vi "Actor Core.vi"(8 "error in":errorcluster, 11 "RecipeEditor in":refnum<class "RecipeEditor.lvclass">) -> (0 "error out":errorcluster, 3 "Actor out":refnum<class "Actor.lvclass">)   [LabVIEW 2024, in "RED Actor.lvlib" / "RecipeEditor.lvclass"]
doc: "(<B>Filename</B>: Actor Framework.lvlib:Actor.lvclass:Actor Core.vi)\n\nReceives messages to the actor, reacts to them, and initiates any error handling that may shut the actor down.\n\nDescendant classes may override this VI to append parallel tasks for the actor to complete while it handles messages. Overrides use the Call Parent Method node."
uses:
  RecipeEditor.lvclass
  C:/Program Files (x86)/National Instruments/LabVIEW 2024/vi.lib/ActorFramework/Actor/Actor.lvclass
  <vilib>/ActorFramework/Actor/Actor.lvclass
  Recipe.ctl
  Setting.ctl
  RedUiStatus.ctl
  RedFunc.ctl
  RecipeEditor.lvclass/RecipeEditor.ctl
  <vilib>/ActorFramework/Actor/Actor.lvclass/Actor.ctl
  <vilib>/ActorFramework/Message Enqueuer/Message Enqueuer.lvclass/Message Enqueuer.ctl
  <vilib>/ActorFramework/Message Enqueuer/Init from Existing Queue.vi
  <vilib>/ActorFramework/Message Enqueuer/Enqueue.vi
  <vilib>/ActorFramework/Stop Msg/Stop Msg.lvclass
  C:/Program Files (x86)/National Instruments/LabVIEW 2024/vi.lib/ActorFramework/Message/Message.lvclass
  Global Variables.vi
  <vilib>/ActorFramework/Message Priority Queue/Priority Enqueue.vi
  <vilib>/ActorFramework/Message Enqueuer/Message Enqueuer.lvclass
panel:
  in  "ExitEdit Button":bool
  out "UIStatus":T1
  in  "Setting Button":bool
  in  "Exit Button":bool
  in  "Save Button":bool
  in  "Upload Button":bool
  in  "Tab Control":enum32{"Recipe", "SystemSetting"}(tab)
  out "DriveWaveform":waveform(dbl)(graph)
  out "LoadWaveform":waveform(dbl)(graph)
  in  "RcpContent":T2={"LoadSide"={"LoadType"=enum."11kW Servo Motor", "LoadMode"=enum."Sin Wave", "LoadValue"=0.0, "PID"={"NP"=0.0, "NI"=0.0, "ND"=0.0, "NPS"="A", "NIS"="A", "NDS"="A"}, "SinWaveFormat"={"Crest"=0.0, "Trugh"=0.0, "Period"=0.0}}, "DriveSide"={"TestSpeed"=0.0, "SinWaveTorqueOutput"=FALSE, "SinWaveFormat"={"Crest"=0.0, "Trugh"=0.0, "Period"=0.0}}} {"DriveSide"."SinWaveFormat"."Period" min=0.0 max=99.0 format="%#.2f"; "DriveSide"."SinWaveFormat"."Trugh" min=0.0 max=99.0 step=1.0 format="%#.2f"; "DriveSide"."SinWaveFormat"."Crest" min=0.0 max=99.0 format="%#.2f"; "DriveSide"."TestSpeed" format="%#_2f"; "LoadSide"."SinWaveFormat"."Period" min=0.0 max=99.0 format="%#.2f"; "LoadSide"."SinWaveFormat"."Trugh" min=0.0 max=99.0 step=1.0 format="%#.2f"; "LoadSide"."SinWaveFormat"."Crest" min=0.0 max=99.0 format="%#.2f"; "LoadSide"."PID"."ND" min=0.0 max=99.0 format="%#.2f"; "LoadSide"."PID"."NI" min=0.0 max=99.0 step=1.0 format="%#.2f"; "LoadSide"."PID"."NP" min=0.0 max=99.0 format="%#.2f"; "LoadSide"."LoadValue" format="%#_2f"}
  in  "Search Button":bool
  in  "SearchingRcp":string
  in  "RecipeList":i32(listbox) caption="參數列表(*.rcp)"
  in  "RecipeFolder":path caption="參數資料夾路徑"
  in  "ButtonContainer":enum32{"Page 1", "Page 2"}(tab)
  in  "Add Button":bool
  in  "Remove Button":bool
  in  "Copy Button":bool
  in  "Modify Button":bool
  in  "TQCalib":bool
  in  "Setting":T3={"TorqueSensor"={"Interface"="", "Read Unit"=enum."Kg.cm", "Encoder"=0, "Torque Filter"=0, "Max Torque"=2.0, "Max Power"=50.0, "Max Speed"=50.0, "Scale Factor CW"=2.0, "Scale Factor CCW"=2.0, "Scale Factor Zero"=2.0}, "DC-1000"={"Interface"=enum."AD-1"}, "ServoMotor"={"Interface"=enum."AD-1"}} {"TorqueSensor"."Scale Factor Zero" format="%#.6f"; "TorqueSensor"."Scale Factor CCW" format="%#.6f"; "TorqueSensor"."Scale Factor CW" format="%#.6f"; "TorqueSensor"."Torque Filter" items=["OFF", "10Hz", "25Hz", "50Hz", "3Hz", "2Hz", "1Hz"]; "TorqueSensor"."Encoder" items=["60-ppr"=60, "600-ppr"=600, "6000-ppr"=6000, "8192-ppr"=8192, "20-ppr"=20, "30-ppr"=30, "1-ppr"=1, "2-ppr"=2, "6-ppr"=6]}
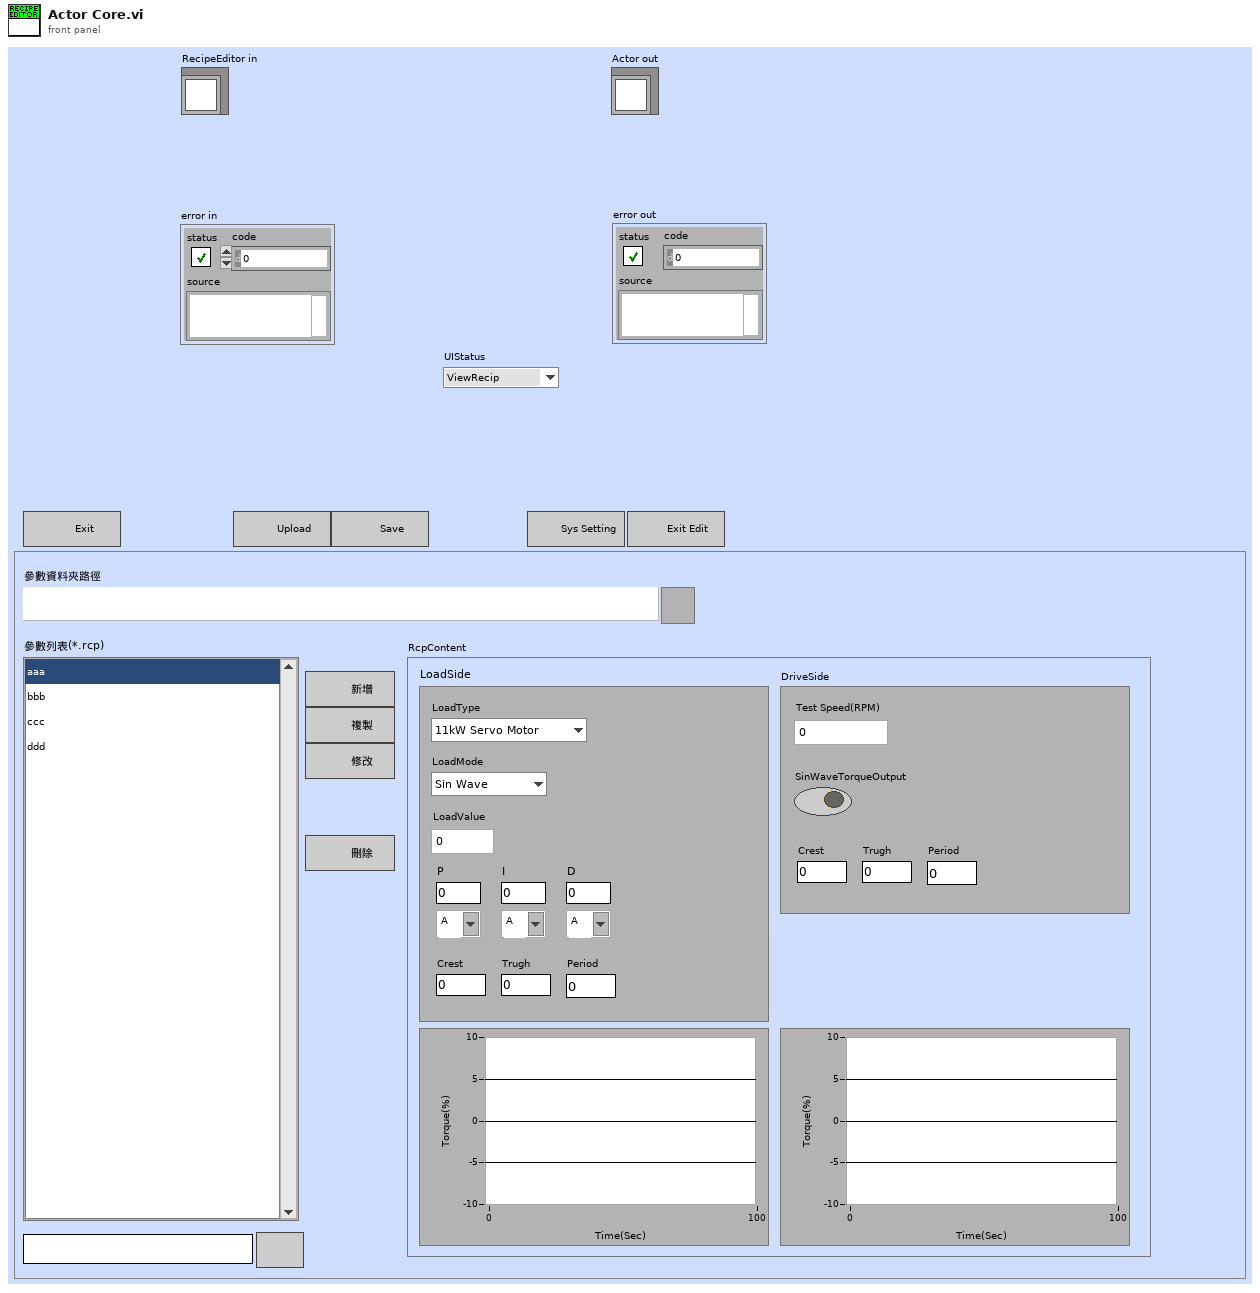
[diagram p1: front panel]
types:
  T1 = typedef "RedUiStatus.ctl" = enum16{"ViewRecip", "EditingRcp", "EditingSet"}
  T2 = typedef "Recipe.ctl" = cluster{"LoadSide":cluster{"LoadType":enum16{"11kW Servo Motor", "Brake"}, "LoadMode":enum16{"Sin Wave", "Torque", "Torque(%)"}, "LoadValue":dbl, "PID":cluster{"NP":dbl, "NI":dbl, "ND":dbl, "NPS":string, "NIS":string, "NDS":string}, "SinWaveFormat":cluster{"Crest":dbl, "Trugh":dbl, "Period":dbl}}, "DriveSide":cluster{"TestSpeed":dbl, "SinWaveTorqueOutput":bool, "SinWaveFormat":cluster{"Crest":dbl, "Trugh":dbl, "Period":dbl}}}
  T3 = typedef "Setting.ctl" = cluster{"TorqueSensor":cluster{"Interface":refnum<visa-resource-name>, "Read Unit":enum16{"oz.in", "oz.ft", "lb.in", "lb.ft", "g.cm", "Kg.cm", "mN.m", "cN.m", "N.m"}, "Encoder":u16, "Torque Filter":u16, "Max Torque":dbl, "Max Power":dbl, "Max Speed":dbl, "Scale Factor CW":dbl, "Scale Factor CCW":dbl, "Scale Factor Zero":dbl}, "DC-1000":cluster{"Interface":enum16{"AD-0", "AD-1"}}, "ServoMotor":cluster{"Interface":enum16{"AD-0", "AD-1"}}}
  T4 = typedef "RedFunc.ctl" = enum16{"None", "InitRED", "LoadRecipes", "UpdateRcpListBtnSts", "ReadRecipe", "RefreshRcpContentUI", "WriteRecipe", "NewRcpFile", "DupRcpFile", "DeleteRcpFile", "Exit"}
  T5 = enum8{"Enabled", "Disabled", "Disabled and Grayed Out"}
  T6 = enum16{"open", "replace", "create", "open or create", "replace or create", "replace or create with confirmation"}
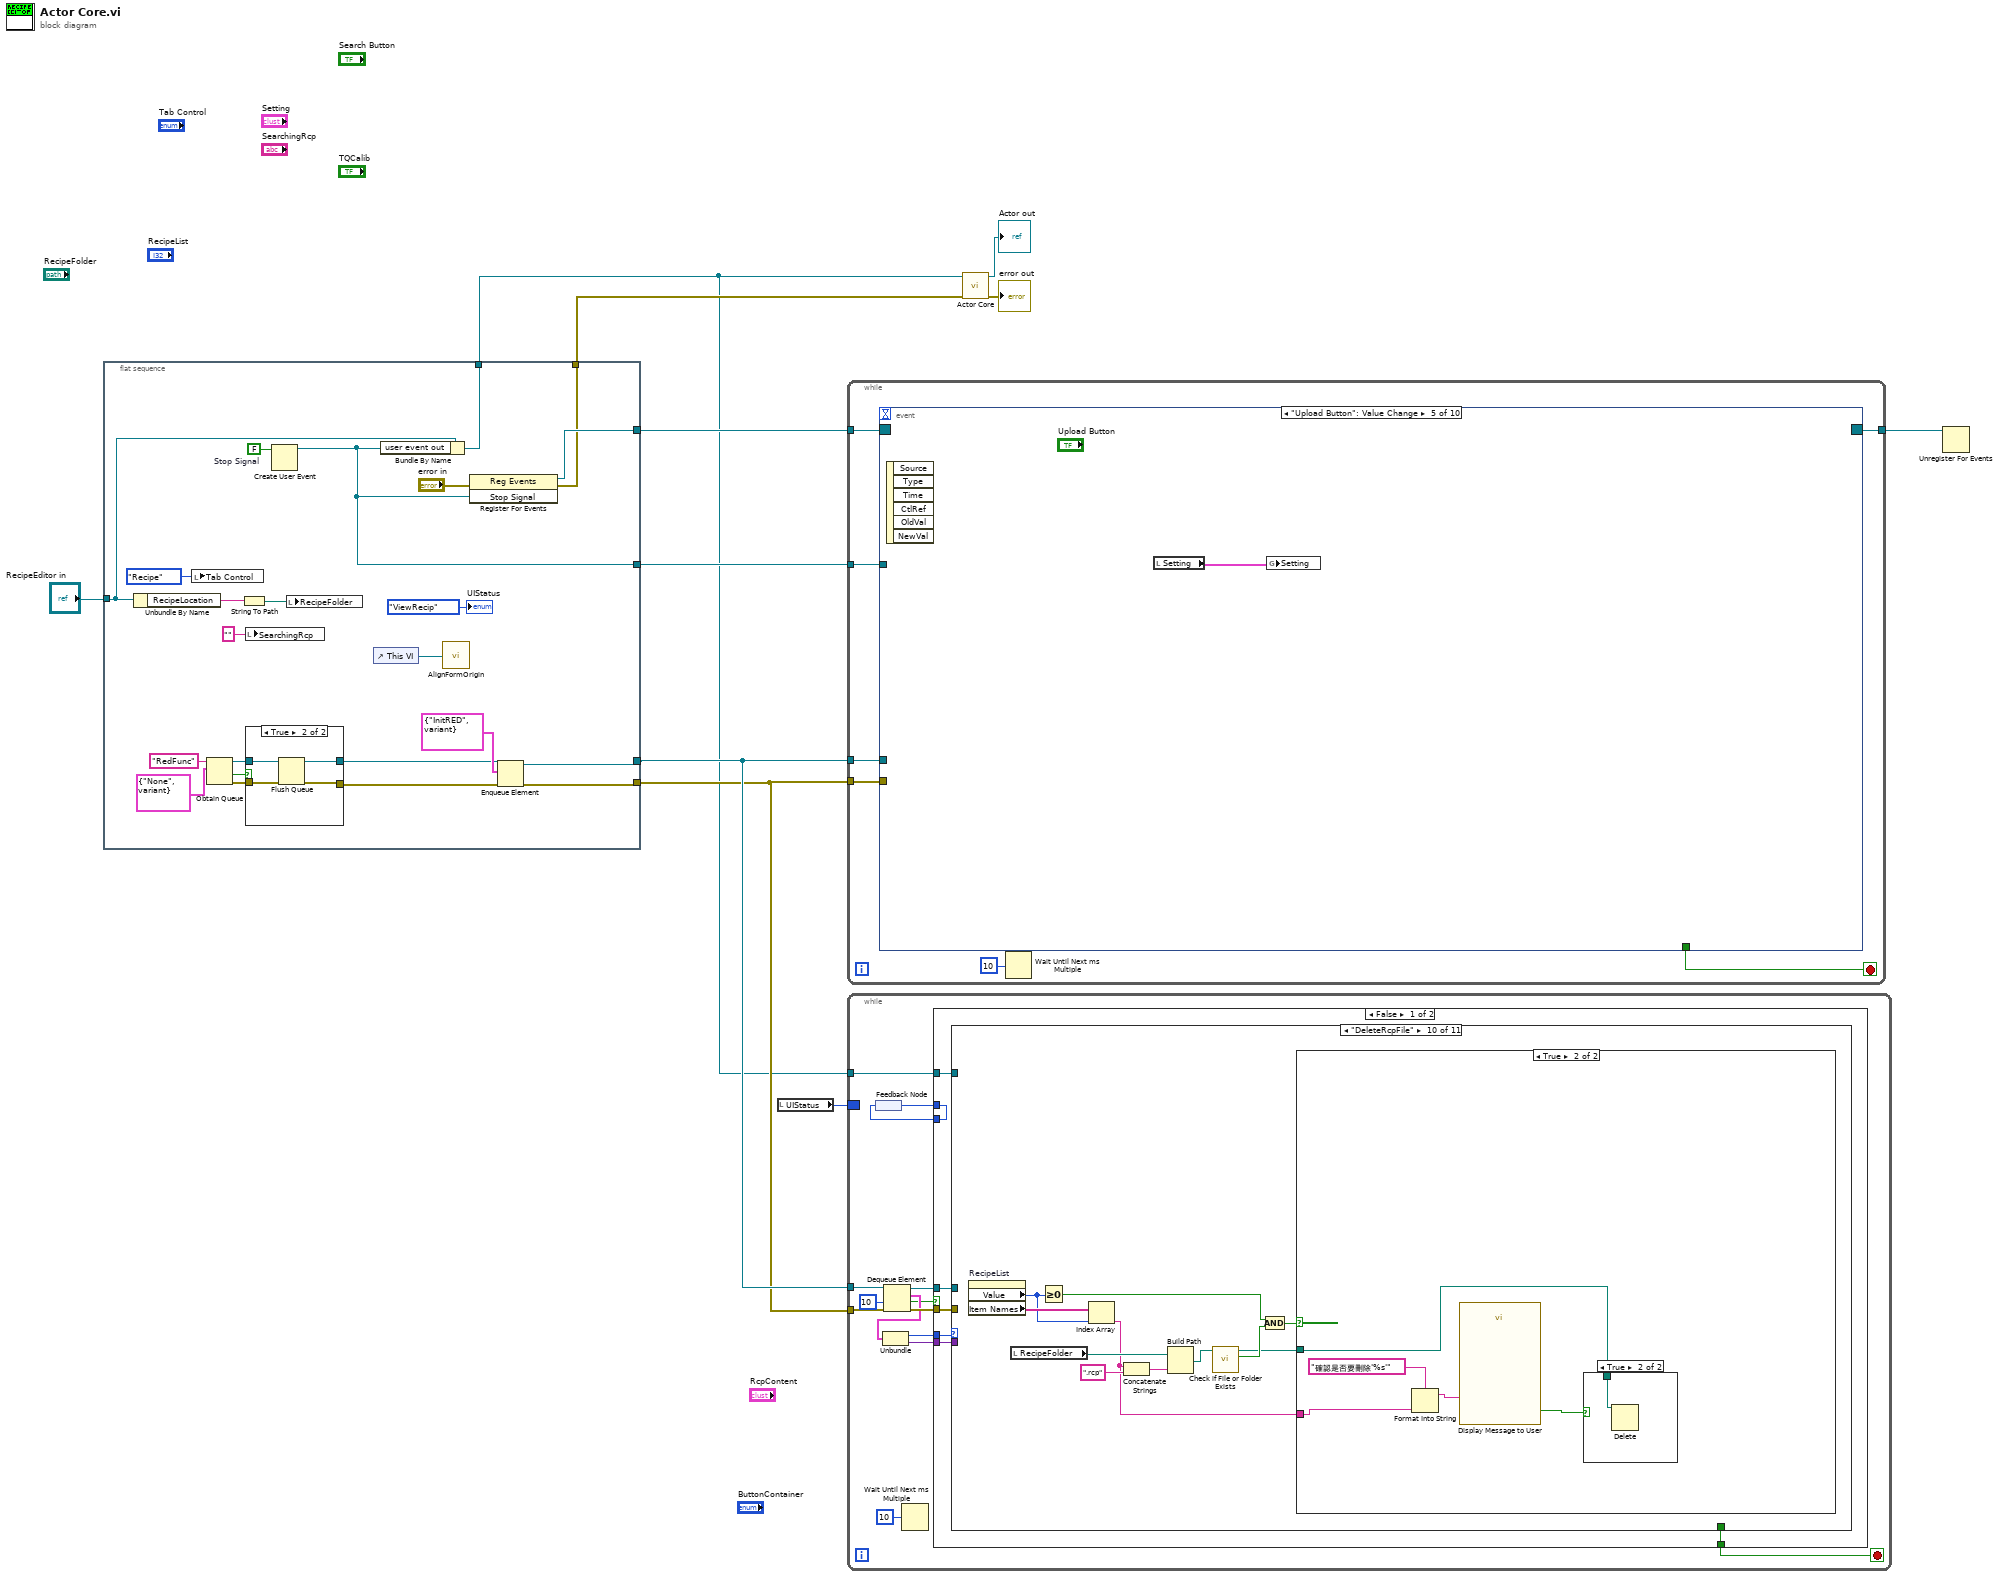
[diagram p0: block diagram]
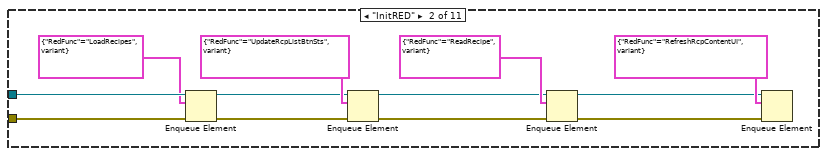
[diagram p4: hidden frame]
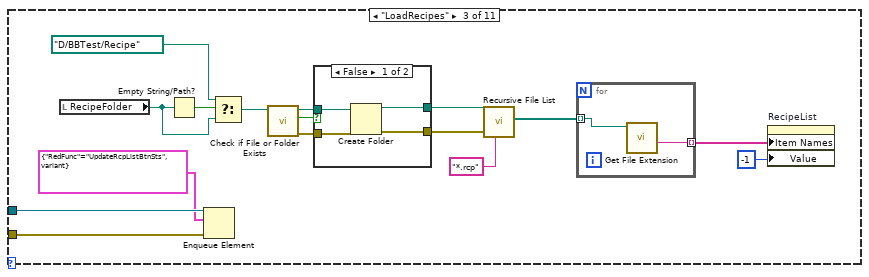
[diagram p5: hidden frame]
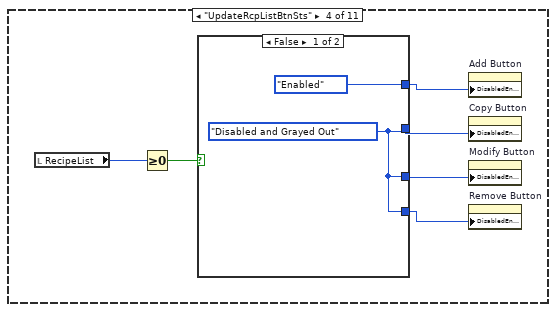
[diagram p7: hidden frame]
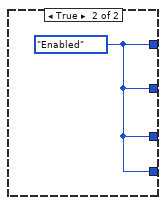
[diagram p8: hidden frame]
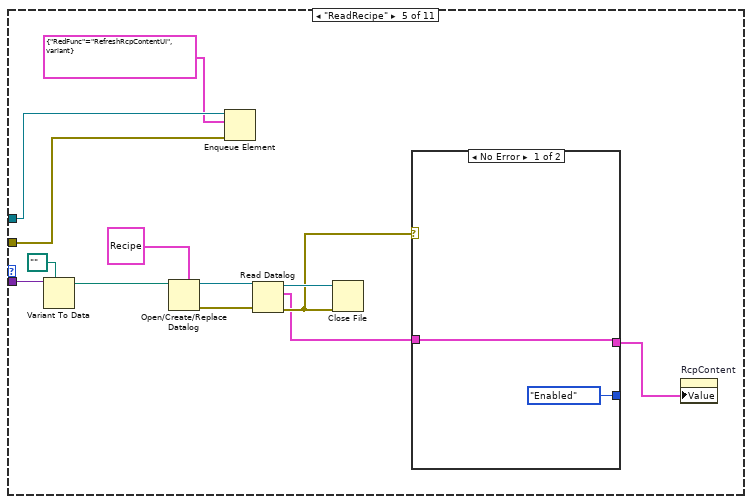
[diagram p9: hidden frame]
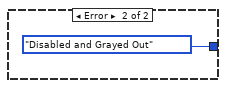
[diagram p10: hidden frame]
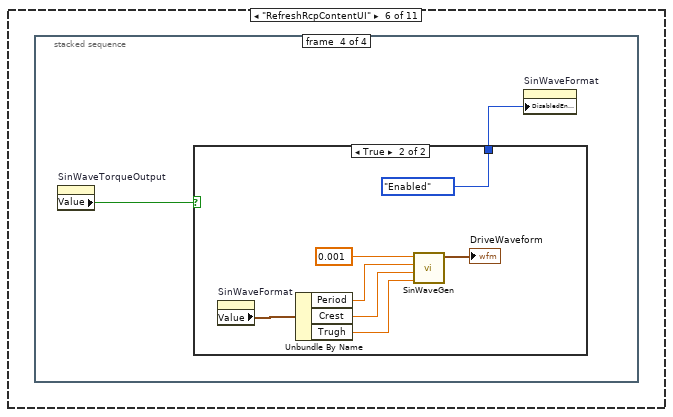
[diagram p11: hidden frame]
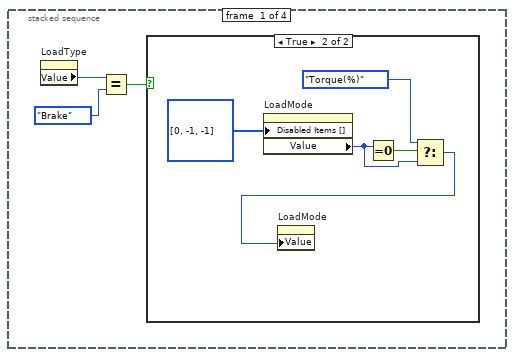
[diagram p12: hidden frame]
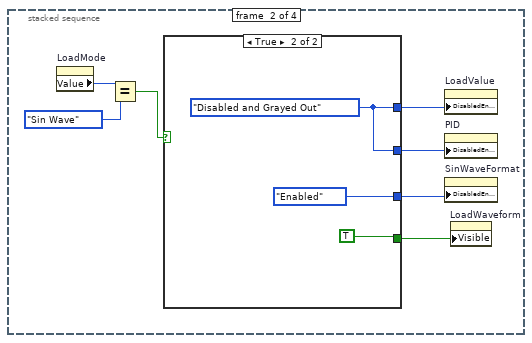
[diagram p14: hidden frame]
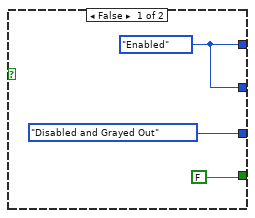
[diagram p15: hidden frame]
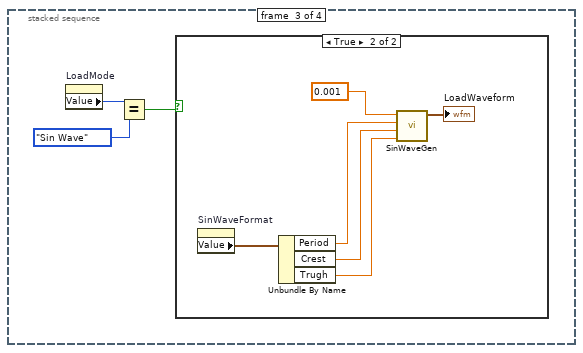
[diagram p16: hidden frame]
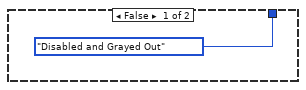
[diagram p18: hidden frame]
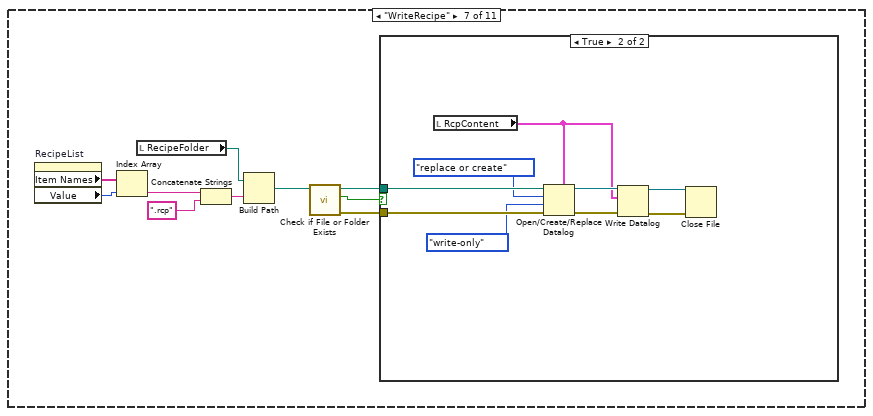
[diagram p19: hidden frame]
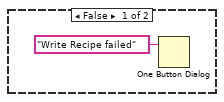
[diagram p20: hidden frame]
diagram:
  n1 = flat-sequence {
    tunnel: "RecipeEditor in" -> [w33]
    tunnel: [w32] -> w1
    tunnel: [w30] -> w8
    tunnel: [w27] -> w6
    tunnel: [w16] -> w5
    tunnel: [w14] -> w4
    tunnel: [w13] -> w3
    frame #0 {
      w34 = FALSE  # Stop Signal
      n2 = Unbundle By Name(w33) -> ("RecipeLocation"=w29:string)
      n3 = local write "Tab Control"(enum32{"Recipe", "SystemSetting"}."Recipe" ("Tab Control")) -> ()
      n4 = Obtain Queue(name (unnamed)="RedFunc", element data type=cluster{"RedFunc":T4, variant} {"RedFunc"=enum."None", variant}) -> (queue out=w24:refnum<queue>, created new?=w23:bool, error out=w25:errorcluster)  [unwired: 3 in]
      n5 = String To Path(string=w29) -> (path=w28:path)
      n6 = local write "SearchingRcp"("" ("SearchingRcp")) -> ()
      n7 = case shown="True" w23 {
        tunnel: w24 -> [w36 w40]
        tunnel: w25 -> [w35 w39]
        tunnel: [w36 w38] -> w17
        tunnel: [w35 w37] -> w15
        frame False {
        }
        frame True {
          n8 = Flush Queue(queue=w40, error in (no error)=w39) -> (queue out=w38:refnum<queue>, error out=w37:errorcluster)  [unwired: 1 out]
        }
      }
      n9 = Create User Event(user event datatype=w34) -> (user event=w13:refnum<user-event>)  [unwired: 1 in, 1 out]
      n10 = local write "RecipeFolder"(w28) -> ()
      n11 = control-ref of="This VI"() -> (w12:refnum<vi>)
      n12 = Bundle By Name(cluster=w33, "user event out"=w13) -> (w32:refnum<class "RecipeEditor.lvclass">)
      n13 = call "AlignFormOrigin.vi"("This VI"=w12) -> ()
      n14 = register-events(error in="error in", w13) -> (reference out=w30:refnum<event-registration>, error out=w27:errorcluster)  [unwired: 1 in]
      n15 = Enqueue Element(queue=w17, element=cluster{"RedFunc":T4, variant} {"RedFunc"=enum."InitRED", variant}, error in (no error)=w15) -> (queue out=w16:refnum<queue>, error out=w14:errorcluster)  [unwired: 1 in, 1 out]
      "UIStatus" <- RedUiStatus."ViewRecip" ("UIStatus")
    }
  }
  n16 = local read "UIStatus"() -> (w2:T1)
  n17 = while {
    tunnel: w8 -> [w47]
    tunnel: [w46] -> w7
    tunnel: w5 -> [w44]
    tunnel: w4 -> [w43]
    tunnel: w3 -> [w42]
    stop <- w45 stop-if-true
    n18 = event shown="[4] \"Upload Button\": Value Change" {
      selector: w47 -> [_ _ _ _ _ _ _ _ _ _]
      dyn-events: [_ _ _ _ _ _ _ _ _ _] -> w46
      timeout: _ -> [_ _ _ _ _ _ _ _ _ _]
      tunnel: [_ TRUE _ _ _ _ _ _ _ _] -> w45
      tunnel: w44 -> [_ w50 w69 _ _ w75 _ _ w85 _]
      tunnel: w43 -> [_ w49 w68 _ _ w74 _ _ w84 _]
      tunnel: w42 -> [_ _ _ w71 _ _ _ _ _ _]
      event Timeout {
        n19 = event-data() -> ()  [unwired: 1 in, 3 out]
      }
      event User Event {
        n20 = event-data() -> ()  [unwired: 1 in, 5 out]
        n21 = Enqueue Element(queue=w50, element=cluster{"RedFunc":T4, variant} {"RedFunc"=enum."Exit", variant}, error in (no error)=w49) -> ()  [unwired: 1 in, 3 out]
      }
      event "RecipeList": Value Change {
        n22 = event-data() -> ("CtlRef"=w62:refnum<vi>, "NewVal"=w63:i32)  [unwired: 1 in, 4 out]
        n23 = property class="LstBox (strict)"(reference=w62) -> ("Item Names"=w61:string[])  [unwired: 1 in, 2 out]
        n24 = Enqueue Element(queue=w69, element=cluster{"RedFunc":T4, variant} {"RedFunc"=enum."UpdateRcpListBtnSts", variant}, error in (no error)=w68) -> (queue out=w66:refnum<queue>, error out=w65:errorcluster)  [unwired: 1 in, 1 out]
        n25 = local read "RecipeFolder"() -> (w64:path)
        n26 = Index Array(array=w61, index=w63) -> (element=w60:string)
        n27 = Concatenate Strings(w60, ".rcp") -> (w58:string)
        n28 = Build Path(base path=w64, name or relative path=w58) -> (appended path=w56:path)
        n29 = Bundle("RedFunc"=RedFunc."ReadRecipe", "appended path"=w56) -> (w55:cluster{"RedFunc":T4, "appended path":path})  [unwired: 1 in]
        n30 = Enqueue Element(queue=w66, element=w55, error in (no error)=w65) -> (queue out=w54:refnum<queue>, error out=w53:errorcluster)  [unwired: 1 in, 1 out]
        n31 = Enqueue Element(queue=w54, element=cluster{"RedFunc":T4, variant} {"RedFunc"=enum."RefreshRcpContentUI", variant}, error in (no error)=w53) -> ()  [unwired: 1 in, 3 out]
      }
      event "Exit Button": Value Change {
        n32 = event-data() -> ()  [unwired: 1 in, 6 out]
        n33 = Generate User Event(user event=w71, event data cluster=TRUE) -> ()  [unwired: 2 in, 2 out]
      }
      event "Upload Button": Value Change {
        n34 = event-data() -> ()  [unwired: 1 in, 6 out]
        n35 = local read "Setting"() -> (w72:T3)
        n36 = global write "Global Variables.vi" "Setting"(w72) -> ()
      }
      event "Save Button": Value Change {
        n37 = event-data() -> ()  [unwired: 1 in, 6 out]
        n38 = Enqueue Element(queue=w75, element=cluster{"RedFunc":T4, variant} {"RedFunc"=enum."WriteRecipe", variant}, error in (no error)=w74) -> ()  [unwired: 1 in, 3 out]
      }
      event "Setting Button": Value Change {
        n39 = event-data() -> ()  [unwired: 1 in, 6 out]
        n40 = local write "Tab Control"(enum32{"Recipe", "SystemSetting"}."SystemSetting" ("Tab Control")) -> ()
        n41 = local write "UIStatus"(RedUiStatus."EditingSet" ("UIStatus")) -> ()
      }
      event "ExitEdit Button": Value Change {
        n42 = event-data() -> ()  [unwired: 1 in, 6 out]
        n43 = local write "Tab Control"(enum32{"Recipe", "SystemSetting"}."Recipe" ("Tab Control")) -> ()
        n44 = local write "UIStatus"(RedUiStatus."ViewRecip" ("UIStatus")) -> ()
      }
      event "Add Button", "Copy Button", "Remove Button": Value Change {
        n45 = event-data() -> ("CtlRef"=w87:refnum<vi>)  [unwired: 1 in, 5 out]
        n46 = property class="Bool"(reference=w87) -> ("Label.Text"=w86:string)  [unwired: 1 in, 2 out]
        n47 = case shown="\"Remove Button\"" w86 {
          tunnel: [cluster{"RedFunc":T4, variant} {"RedFunc"=enum."NewRcpFile", variant} cluster{"RedFunc":T4, variant} {"RedFunc"=enum."DupRcpFile", variant} cluster{"RedFunc":T4, variant} {"RedFunc"=enum."DeleteRcpFile", variant}] -> w83
          frame "Add Button", Default {
          }
          frame "Copy Button" {
          }
          frame "Remove Button" {
          }
        }
        n48 = Enqueue Element(queue=w85, element=w83, error in (no error)=w84) -> (queue out=w82:refnum<queue>, error out=w81:errorcluster)  [unwired: 1 in, 1 out]
        n49 = Enqueue Element(queue=w82, element=cluster{"RedFunc":T4, variant} {"RedFunc"=enum."LoadRecipes", variant}, error in (no error)=w81) -> ()  [unwired: 1 in, 3 out]
      }
      event "Modify Button": Value Change {
        n50 = event-data() -> ()  [unwired: 1 in, 6 out]
        n51 = local write "UIStatus"(RedUiStatus."EditingRcp" ("UIStatus")) -> ()
      }
    }
    n52 = Wait Until Next ms Multiple(millisecond multiple=u32 10) -> ()  [unwired: 1 out]
  }
  n53 = while {
    tunnel: w5 -> [w105]
    tunnel: w4 -> [w104]
    border: w2 -> [_]
    tunnel: w1 -> [w92]
    stop <- w98 stop-if-true
    n54 = feedback #1() -> (w94:T1)
    n55 = Dequeue Element(queue=w105, timeout in ms (-1)=10, error in (no error)=w104) -> (queue out=w103:refnum<queue>, element=w101:cluster{"RedFunc":T4, variant}, timed out?=w95:bool, error out=w102:errorcluster)
    n56 = Unbundle(w101) -> ("RedFunc"=w100:T4, w99:variant)
    n57 = Wait Until Next ms Multiple(millisecond multiple=u32 10) -> ()  [unwired: 1 out]
    n58 = case shown="False" w95 {
      tunnel: w103 -> [w112 _]
      tunnel: w102 -> [w111 _]
      tunnel: w100 -> [w110 _]
      tunnel: w99 -> [w109 _]
      tunnel: [w108 _] -> w98
      tunnel: w94 -> [w107 w339]
      tunnel: [w107 w335] -> w93
      tunnel: w92 -> [w106 _]
      frame False {
        n59 = case shown="\"DeleteRcpFile\"" w110 {
          tunnel: w112 -> [_ w124 w127 _ w160 _ _ _ _ _ w333]
          tunnel: w111 -> [_ w123 w126 _ w159 _ _ _ _ _ w332]
          tunnel: w109 -> [_ _ _ _ w170 _ _ _ _ _ _]
          tunnel: [_ _ _ _ _ _ _ _ _ _ TRUE] -> w108
          tunnel: w106 -> [_ _ _ _ _ _ _ _ _ _ w329]
          frame "None", Default {
          }
          frame "InitRED" {
            n60 = Enqueue Element(queue=w124, element=cluster{"RedFunc":T4, variant} {"RedFunc"=enum."LoadRecipes", variant}, error in (no error)=w123) -> (queue out=w120:refnum<queue>, error out=w119:errorcluster)  [unwired: 1 in, 1 out]
            n61 = Enqueue Element(queue=w120, element=cluster{"RedFunc":T4, variant} {"RedFunc"=enum."UpdateRcpListBtnSts", variant}, error in (no error)=w119) -> (queue out=w117:refnum<queue>, error out=w116:errorcluster)  [unwired: 1 in, 1 out]
            n62 = Enqueue Element(queue=w117, element=cluster{"RedFunc":T4, variant} {"RedFunc"=enum."ReadRecipe", variant}, error in (no error)=w116) -> (queue out=w114:refnum<queue>, error out=w113:errorcluster)  [unwired: 1 in, 1 out]
            n63 = Enqueue Element(queue=w114, element=cluster{"RedFunc":T4, variant} {"RedFunc"=enum."RefreshRcpContentUI", variant}, error in (no error)=w113) -> ()  [unwired: 1 in, 3 out]
          }
          frame "LoadRecipes" {
            n64 = local read "RecipeFolder"() -> (w136:path)
            n65 = Empty String/Path?(string/path=w136) -> (empty?=w137:bool)
            n66 = Enqueue Element(queue=w127, element=cluster{"RedFunc":T4, variant} {"RedFunc"=enum."UpdateRcpListBtnSts", variant}, error in (no error)=w126) -> ()  [unwired: 1 in, 3 out]
            n67 = Select(t=path "D:/BBTest/Recipe", s=w137, f=w136) -> (s? t:f=w135:path)
            n68 = call <vilib>:"Check if File or Folder Exists.vi"("path"=w135) -> ("error out"=w138:errorcluster, "file or folder exists?"=w140:bool, "dup path"=w139:path)  [unwired: 8 in]
            n69 = case shown="False" w140 {
              tunnel: w139 -> [w146 w148]
              tunnel: w138 -> [w145 w147]
              tunnel: [w144 w148] -> w133
              tunnel: [w143 w147] -> w132
              frame False {
                n70 = Create Folder(path (use dialog)=w146, error in=w145) -> (created path=w144:path, error out=w143:errorcluster)  [unwired: 1 in, 1 out]
              }
              frame True {
              }
            }
            n71 = call <vilib>:"Recursive File List.vi"("pattern"="*.rcp", "error in (no error)"=w132, "Folder Path"=w133) -> ("All Files in Dir"=w130:path[])  [unwired: 4 in, 4 out]
            n72 = for {
              tunnel: w130 -> [w142] mode=indexing
              tunnel: [w141] -> w129 mode=indexing
              n73 = call <vilib>:"Get File Extension.vi"("file"=w142) -> ("filename without extension"=w141:string)  [unwired: 6 in, 4 out]
            }
            n74 = property on="RecipeList" class="LstBox (strict)"("Item Names"=w129, "Value"=-1 ("Value (Signaling)")) -> ()  [unwired: 2 in, 2 out]
          }
          frame "UpdateRcpListBtnSts" {
            n75 = local read "RecipeList"() -> (w154:i32)
            n76 = Greater Or Equal To 0?(x=w154) -> (x >= 0?=w153:bool)
            n77 = case shown="False" w153 {
              tunnel: [T5."Enabled" ("Disabled") w157] -> w152
              tunnel: [w155 w157] -> w151
              tunnel: [w155 w157] -> w150
              tunnel: [w155 w157] -> w149
              frame False {
                w155 = T5."Disabled and Grayed Out" ("Disabled")
              }
              frame True {
                w157 = T5."Enabled" ("Disabled")
              }
            }
            n78 = property on="Add Button" class="Bool"("DisabledEnum"=w152) -> ()  [unwired: 2 in, 2 out]
            n79 = property on="Copy Button" class="Bool"("DisabledEnum"=w151) -> ()  [unwired: 2 in, 2 out]
            n80 = property on="Modify Button" class="Bool"("DisabledEnum"=w150) -> ()  [unwired: 2 in, 2 out]
            n81 = property on="Remove Button" class="Bool"("DisabledEnum"=w149) -> ()  [unwired: 2 in, 2 out]
          }
          frame "ReadRecipe" {
            n82 = Variant To Data(type=path "", Variant=w170) -> (data=w168:path)  [unwired: 1 in, 1 out]
            n83 = Open/Create/Replace Datalog(5:T2 {"LoadSide"={"LoadType"=enum."11kW Servo Motor", "LoadMode"=enum."Sin Wave", "LoadValue"=0.0, "PID"={"NP"=0.0, "NI"=0.0, "ND"=0.0, "NPS"="A", "NIS"="A", "NDS"="A"}, "SinWaveFormat"={"Crest"=0.0, "Trugh"=0.0, "Period"=0.0}}, "DriveSide"={"TestSpeed"=0.0, "SinWaveTorqueOutput"=FALSE, "SinWaveFormat"={"Crest"=0.0, "Trugh"=0.0, "Period"=0.0}}} ("RcpContent"), 11:w168) -> (0:w165:errorcluster, 3:w166:refnum<k1>)  [unwired: 4 in, 1 out]
            n84 = Enqueue Element(queue=w160, element=cluster{"RedFunc":T4, variant} {"RedFunc"=enum."RefreshRcpContentUI", variant}, error in (no error)=w159) -> ()  [unwired: 1 in, 3 out]
            n85 = Read Datalog(4:w165, 7:w166) -> (0:w163:errorcluster, 2:w162:T2, 3:w164:refnum<k1>)  [unwired: 1 in]
            n86 = Close File(refnum=w164, error in=w163) -> ()  [unwired: 2 out]
            n87 = case shown="No Error" w163 {
              tunnel: w162 -> [w172 _]
              tunnel: [w172 _] -> w161
              tunnel: [T5."Enabled" ("Disabled") T5."Disabled and Grayed Out" ("Disabled")] -> _
              frame No Error {
              }
              frame Error {
              }
            }
            n88 = property on="RcpContent" class="Clust (strict)"("Value"=w161) -> ()  [unwired: 2 in, 2 out]
          }
          frame "RefreshRcpContentUI" {
            n89 = stacked-sequence {
              frame #0 {
                n90 = property on="LoadType" class="Enum (strict)"() -> ("Value"=w176:enum16{"11kW Servo Motor", "Brake"})  [unwired: 2 in, 2 out]
                n91 = Equal?(x=w176, y=enum16{"11kW Servo Motor", "Brake"}."Brake" ("Value")) -> (x = y?=w174:bool)
                n92 = case shown="True" w174 {
                  frame False {
                  }
                  frame True {
                    n93 = property on="LoadMode" class="Enum (strict)"("Disabled Items []"=i32[] [0, -1, -1]) -> ("Value"=w178:enum16{"Sin Wave", "Torque", "Torque(%)"})  [unwired: 2 in, 2 out]
                    n94 = Equal To 0?(x=w178) -> (x = 0?=w180:bool)
                    n95 = Select(t=enum16{"Sin Wave", "Torque", "Torque(%)"}."Torque(%)" ("Value"), s=w180, f=w178) -> (s? t:f=w177:enum16{"Sin Wave", "Torque", "Torque(%)"})
                    n96 = property on="LoadMode" class="Enum (strict)"("Value"=w177) -> ()  [unwired: 2 in, 2 out]
                  }
                }
              }
              frame #1 {
                n97 = property on="LoadMode" class="Enum (strict)"() -> ("Value"=w188:enum16{"Sin Wave", "Torque", "Torque(%)"})  [unwired: 2 in, 2 out]
                n98 = Equal?(x=w188, y=enum16{"Sin Wave", "Torque", "Torque(%)"}."Sin Wave") -> (x = y?=w186:bool)
                n99 = case shown="True" w186 {
                  tunnel: [w190 w194] -> w185
                  tunnel: [w190 w194] -> w184
                  tunnel: [T5."Disabled and Grayed Out" ("Disabled") T5."Enabled" ("Disabled")] -> w183
                  tunnel: [FALSE TRUE] -> w182
                  frame False {
                    w190 = T5."Enabled" ("Disabled")
                  }
                  frame True {
                    w194 = T5."Disabled and Grayed Out" ("Disabled")
                  }
                }
                n100 = property on="LoadValue" class="DigNum (strict)"("DisabledEnum"=w185) -> ()  [unwired: 2 in, 2 out]
                n101 = property on="PID" class="Clust (strict)"("DisabledEnum"=w184) -> ()  [unwired: 2 in, 2 out]
                n102 = property on="SinWaveFormat" class="Clust (strict)"("DisabledEnum"=w183) -> ()  [unwired: 2 in, 2 out]
                n103 = property on="LoadWaveform" class="WFGraph (strict)"("Visible"=w182) -> ()  [unwired: 2 in, 2 out]
              }
              frame #2 {
                n104 = property on="LoadMode" class="Enum (strict)"() -> ("Value"=w197:enum16{"Sin Wave", "Torque", "Torque(%)"})  [unwired: 2 in, 2 out]
                n105 = Equal?(x=w197, y=enum16{"Sin Wave", "Torque", "Torque(%)"}."Sin Wave") -> (x = y?=w195:bool)
                n106 = case shown="True" w195 {
                  frame False {
                  }
                  frame True {
                    n107 = property on="SinWaveFormat" class="Clust (strict)"() -> ("Value"=w202:cluster{"Crest":dbl, "Trugh":dbl, "Period":dbl})  [unwired: 2 in, 2 out]
                    n108 = Unbundle By Name(w202) -> ("Period"=w201:dbl, "Crest"=w199:dbl, "Trugh"=w200:dbl)
                    n109 = call "SinWaveGen.vi"("WaveTrough"=w200, "WaveCrest"=w199, "SinWavePeriod(Sec)"=w201, "dt"=0.001) -> ("Waveform"=→"LoadWaveform":waveform(dbl))  [unwired: 6 in, 1 out]
                  }
                }
              }
              frame #3 {
                n110 = property on="SinWaveTorqueOutput" class="Bool (strict)"() -> ("Value"=w205:bool)  [unwired: 2 in, 2 out]
                n111 = case shown="True" w205 {
                  tunnel: [T5."Disabled and Grayed Out" ("Disabled") T5."Enabled" ("Disabled")] -> w204
                  frame False {
                  }
                  frame True {
                    n112 = property on="SinWaveFormat" class="Clust (strict)"() -> ("Value"=w209:cluster{"Crest":dbl, "Trugh":dbl, "Period":dbl})  [unwired: 2 in, 2 out]
                    n113 = Unbundle By Name(w209) -> ("Period"=w212:dbl, "Crest"=w210:dbl, "Trugh"=w211:dbl)
                    n114 = call "SinWaveGen.vi"("WaveTrough"=w211, "WaveCrest"=w210, "SinWavePeriod(Sec)"=w212, "dt"=0.001) -> ("Waveform"=→"DriveWaveform":waveform(dbl))  [unwired: 6 in, 1 out]
                  }
                }
                n115 = property on="SinWaveFormat" class="Clust (strict)"("DisabledEnum"=w204) -> ()  [unwired: 2 in, 2 out]
              }
            }
          }
          frame "WriteRecipe" {
            n116 = property on="RecipeList" class="LstBox (strict)"() -> ("Item Names"=w220:string[], "Value"=w219:i32)  [unwired: 2 in, 2 out]
            n117 = Index Array(array=w220, index=w219) -> (element=w218:string)
            n118 = local read "RecipeFolder"() -> (w216:path)
            n119 = Concatenate Strings(w218, ".rcp") -> (w215:string)
            n120 = Build Path(base path=w216, name or relative path=w215) -> (appended path=w214:path)
            n121 = call <vilib>:"Check if File or Folder Exists.vi"("path"=w214) -> ("error out"=w221:errorcluster, "file or folder exists?"=w223:bool, "dup path"=w222:path)  [unwired: 8 in]
            n122 = case shown="True" w223 {
              tunnel: w222 -> [_ w233]
              tunnel: w221 -> [_ w232]
              frame False {
                n123 = One Button Dialog(message="Write Recipe failed") -> ()  [unwired: 1 in, 1 out]
              }
              frame True {
                n124 = local read "RcpContent"() -> (w228:T2)
                n125 = Open/Create/Replace Datalog(5:w228, 8:w232, 9:enum16{"read/write", "read-only", "write-only"}."write-only" ("access (0:read/write)"), 10:T6."replace or create" ("operation (0:open)"), 11:w233) -> (0:w229:errorcluster, 3:w230:refnum<k1>)  [unwired: 1 in, 1 out]
                n126 = Write Datalog(4:w229, 6:w228, 7:w230) -> (0:w226:errorcluster, 3:w227:refnum<k1>)
                n127 = Close File(refnum=w227, error in=w226) -> ()  [unwired: 2 out]
              }
            }
          }
          frame "NewRcpFile" {
            n128 = local read "RecipeFolder"() -> (w236:path)
            n129 = call <vilib>:"Check if File or Folder Exists.vi"("path"=w236) -> ("error out"=w234:errorcluster, "file or folder exists?"=w237:bool, "dup path"=w235:path)  [unwired: 8 in]
            n130 = case shown="True" w237 {
              tunnel: w235 -> [_ w242]
              tunnel: w234 -> [_ w241]
              frame False {
              }
              frame True {
                n131 = File/Directory Info(path=w242, error in=w241) -> (path out=w238:path, directory=w240:bool, error out=w239:errorcluster)  [unwired: 4 out]
                n132 = case shown="True" w240 {
                  tunnel: w239 -> [_ w247]
                  tunnel: w238 -> [_ w246]
                  frame False {
                  }
                  frame True {
                    n133 = call "新增參數"("error in (no error)"=w247) -> (17:w245:string, "OK"=w243:bool, "error out"=w244:errorcluster)  [unwired: 16 in]
                    n134 = case shown="True" w243 {
                      tunnel: w246 -> [_ w259]
                      tunnel: w245 -> [_ w250]
                      tunnel: w244 -> [_ w256]
                      frame False {
                      }
                      frame True {
                        n135 = call <vilib>:"Recursive File List.vi"("pattern"="*.rcp", "error in (no error)"=w256, "Folder Path"=w259) -> ("All Files in Dir"=w258:path[], "dup Folder Path"=w253:path)  [unwired: 4 in, 3 out]
                        n136 = for {
                          tunnel: w258 -> [w273] mode=indexing
                          tunnel: [w272] -> _ mode=indexing
                          tunnel: [w271] -> w257 mode=indexing
                          n137 = call <vilib>:"Get File Extension.vi"("file"=w273) -> ("error out"=w272:errorcluster, "filename without extension"=w271:string)  [unwired: 6 in, 3 out]
                        }
                        n138 = Concatenate Strings(w250, ".rcp" ("pattern")) -> (w252:string)
                        n139 = Search 1D Array(1D array=w257, element=w250) -> (index of element=w255:i32)  [unwired: 1 in]
                        n140 = Build Path(base path=w253, name or relative path=w252) -> (appended path=w251:path)
                        n141 = Less Than 0?(x=w255) -> (x < 0?=w254:bool)
                        n142 = case shown="True" w254 {
                          tunnel: w251 -> [_ w265]
                          tunnel: w250 -> [w261 _]
                          frame False {
                            n143 = Format Into String(format string="'%s' is exsisted", w261) -> (resulting string=w260:string)  [unwired: 2 in, 1 out]
                            n144 = One Button Dialog(message=w260) -> ()  [unwired: 1 in, 1 out]
                          }
                          frame True {
                            w263 = T2 {"LoadSide"={"LoadType"=enum."11kW Servo Motor", "LoadMode"=enum."Sin Wave", "LoadValue"=0.0, "PID"={"NP"=0.0, "NI"=0.0, "ND"=0.0, "NPS"="A", "NIS"="A", "NDS"="A"}, "SinWaveFormat"={"Crest"=0.0, "Trugh"=0.0, "Period"=0.0}}, "DriveSide"={"TestSpeed"=0.0, "SinWaveTorqueOutput"=FALSE, "SinWaveFormat"={"Crest"=0.0, "Trugh"=0.0, "Period"=0.0}}} ("RcpContent")
                            n145 = Open/Create/Replace Datalog(5:w263, 9:enum16{"read/write", "read-only", "write-only"}."write-only" ("access (0:read/write)"), 10:T6."replace or create" ("operation (0:open)"), 11:w265) -> (0:w269:errorcluster, 3:w264:refnum<k1>)  [unwired: 2 in, 1 out]
                            n146 = Write Datalog(4:w269, 6:w263, 7:w264) -> (0:w267:errorcluster, 3:w268:refnum<k1>)
                            n147 = Close File(refnum=w268, error in=w267) -> ()  [unwired: 2 out]
                          }
                        }
                      }
                    }
                  }
                }
              }
            }
          }
          frame "DupRcpFile" {
            w275 = ".rcp" ("string")
            n148 = property on="RecipeList" class="LstBox (strict)"() -> ("Value"=w283:i32, "Item Names"=w284:string[])  [unwired: 2 in, 2 out]
            n149 = local read "RecipeFolder"() -> (w274:path)
            n150 = Greater Or Equal To 0?(x=w283) -> (x >= 0?=w278:bool)
            n151 = Index Array(array=w284, index=w283) -> (element=w282:string)
            n152 = Concatenate Strings(w282, w275) -> (w281:string)
            n153 = Build Path(base path=w274, name or relative path=w281) -> (appended path=w280:path)
            n154 = call <vilib>:"Check if File or Folder Exists.vi"("path"=w280) -> ("file or folder exists?"=w279:bool, "dup path"=w276:path)  [unwired: 8 in, 1 out]
            n155 = And(x=w278, y=w279) -> (x .and. y?=w277:bool)
            n156 = case shown="True" w277 {
              tunnel: w276 -> [_ w286]
              tunnel: w275 -> [_ w292]
              tunnel: w274 -> [_ w288]
              frame False {
              }
              frame True {
                n157 = call "複製參數"() -> (17:w289:string, "OK"=w287:bool, "error out"=w290:errorcluster)  [unwired: 17 in]
                n158 = Concatenate Strings(w289, w292) -> (w291:string)
                n159 = Build Path(base path=w288, name or relative path=w291) -> (appended path=w285:path)
                n160 = case shown="True" w287 {
                  tunnel: w290 -> [_ w301]
                  tunnel: w289 -> [w293 w300]
                  tunnel: w288 -> [_ w298]
                  tunnel: w286 -> [_ w297]
                  tunnel: w285 -> [_ w296]
                  frame False {
                    n161 = Format Into String(format string="'%s' is exsisted", w293) -> (resulting string=w294:string)  [unwired: 2 in, 1 out]
                    n162 = One Button Dialog(message=w294) -> ()  [unwired: 1 in, 1 out]
                  }
                  frame True {
                    n163 = call <vilib>:"Recursive File List.vi"("pattern"="*.rcp", "error in (no error)"=w301, "Folder Path"=w298) -> ("All Files in Dir"=w305:path[])  [unwired: 4 in, 4 out]
                    n164 = for {
                      tunnel: w305 -> [w310] mode=indexing
                      tunnel: [w309] -> _ mode=indexing
                      tunnel: [w308] -> w304 mode=indexing
                      n165 = call <vilib>:"Get File Extension.vi"("file"=w310) -> ("error out"=w309:errorcluster, "filename without extension"=w308:string)  [unwired: 6 in, 3 out]
                    }
                    n166 = Search 1D Array(1D array=w304, element=w300) -> (index of element=w303:i32)  [unwired: 1 in]
                    n167 = Less Than 0?(x=w303) -> (x < 0?=w299:bool)
                    n168 = case shown="True" w299 {
                      tunnel: w297 -> [_ w307]
                      tunnel: w296 -> [_ w306]
                      frame False {
                      }
                      frame True {
                        n169 = Copy(10:w306, 11:w307) -> ()  [unwired: 3 in, 3 out]
                      }
                    }
                  }
                }
              }
            }
          }
          frame "DeleteRcpFile" {
            n170 = property on="RecipeList" class="LstBox (strict)"() -> ("Value"=w320:i32, "Item Names"=w321:string[])  [unwired: 2 in, 2 out]
            n171 = local read "RecipeFolder"() -> (w313:path)
            n172 = Greater Or Equal To 0?(x=w320) -> (x >= 0?=w316:bool)
            n173 = Index Array(array=w321, index=w320) -> (element=w311:string)
            n174 = Concatenate Strings(w311, ".rcp" ("string")) -> (w319:string)
            n175 = Build Path(base path=w313, name or relative path=w319) -> (appended path=w318:path)
            n176 = call <vilib>:"Check if File or Folder Exists.vi"("path"=w318) -> ("file or folder exists?"=w317:bool, "dup path"=w314:path)  [unwired: 8 in, 1 out]
            n177 = And(x=w316, y=w317) -> (x .and. y?=w315:bool)
            n178 = case shown="True" w315 {
              tunnel: w314 -> [_ w322]
              tunnel: w311 -> [_ w325]
              frame False {
              }
              frame True {
                n179 = Format Into String(format string="確認是否要刪除'%s'", w325) -> (resulting string=w324:string)  [unwired: 2 in, 1 out]
                n180 = call "Display Message to User"("Message"=w324) -> ("OK"=w323:bool)  [unwired: 9 in, 1 out]
                n181 = case shown="True" w323 {
                  tunnel: w322 -> [_ w327]
                  frame False {
                  }
                  frame True {
                    n182 = Delete(path (use dialog)=w327) -> ()  [unwired: 4 in, 3 out]
                  }
                }
              }
            }
          }
          frame "Exit" {
            n183 = Flush Queue(queue=w333, error in (no error)=w332) -> (queue out=w331:refnum<queue>, error out=w330:errorcluster)  [unwired: 1 out]
            n184 = call <vilib>:"Read Self Enqueuer.vi"("Actor"=w329) -> ("Self Enqueuer"=w328:refnum<class "Message Enqueuer.lvclass">)  [unwired: 10 in]
            n185 = call <vilib>:"Send Normal Stop.vi"("Message Enqueuer"=w328) -> ()  [unwired: 10 in, 1 out]
            n186 = Release Queue(queue=w331, error in (no error)=w330) -> ()  [unwired: 1 in, 3 out]
          }
        }
      }
      frame True {
        n187 = local read "UIStatus"() -> (w335:T1)
        n188 = Not Equal?(x=w339, y=w335) -> (x != y?=w337:bool)
        n189 = First Call?() -> (First Call?: T/F=w338:bool)
        n190 = Or(x=w338, y=w337) -> (x .or. y?=w336:bool)
        n191 = case shown="True" w336 {
          tunnel: w335 -> [_ w342]
          frame False {
          }
          frame True {
            n192 = case shown="\"ViewRecip\", Default" w342 {
              tunnel: [w349 w352 w355] -> w348
              tunnel: [w351 w353 w354] -> w347
              tunnel: [w349 w352 w355] -> _
              tunnel: [w349 w352 w355] -> w346
              tunnel: [w351 w353 w354] -> w345
              tunnel: [w349 w352 w354] -> w344
              tunnel: [T5."Disabled" ("Disabled") w353 T5."Disabled" ("Disabled")] -> w343
              tunnel: [w349 w352 w355] -> w341
              tunnel: [w349 w352 w354] -> w340
              frame "ViewRecip", Default {
                w349 = T5."Enabled" ("Disabled")
                w351 = T5."Disabled and Grayed Out" ("Disabled")
              }
              frame "EditingRcp" {
                w353 = T5."Enabled" ("Disabled")
                w352 = T5."Disabled and Grayed Out" ("Disabled")
              }
              frame "EditingSet" {
                w354 = T5."Enabled" ("Disabled")
                w355 = T5."Disabled and Grayed Out" ("Disabled")
              }
            }
            n193 = property on="RcpContent" class="Clust (strict)"("DisabledEnum"=w343) -> ()  [unwired: 2 in, 2 out]
            n194 = property on="RecipeList" class="LstBox (strict)"("DisabledEnum"=w344) -> ()  [unwired: 2 in, 2 out]
            n195 = property on="Exit Button" class="Bool"("DisabledEnum"=w341) -> ()  [unwired: 2 in, 2 out]
            n196 = property on="Upload Button" class="Bool"("DisabledEnum"=w348) -> ()  [unwired: 2 in, 2 out]
            n197 = property on="Save Button" class="Bool"("DisabledEnum"=w347) -> ()  [unwired: 2 in, 2 out]
            n198 = property on="Setting Button" class="Bool"("DisabledEnum"=w346) -> ()  [unwired: 2 in, 2 out]
            n199 = property on="ExitEdit Button" class="Bool"("DisabledEnum"=w345) -> ()  [unwired: 2 in, 2 out]
            n200 = property on="ButtonContainer" class="TabCtl (strict)"("DisabledEnum"=w340) -> ()  [unwired: 2 in, 2 out]
          }
        }
      }
    }
    n201 = feedback-in #1(w93) -> ()
  }
  n202 = call-parent "Actor Core.vi"("error in"=w6, "Actor in"=w1) -> ("error out"=→"error out":errorcluster, "Actor out"=→"Actor out":refnum<class "Actor.lvclass">)  [unwired: 8 in]
  n203 = Unregister For Events(event registration refnum=w7) -> ()  [unwired: 1 in, 1 out]
